vi "Agilent 34970 Set Switch.vi"(7 "Open/Close (F:Close)":bool, 8 "error in (no error)":errorcluster, 10 "Channel":string, 11 "VISA Refnum in":refnum<visa-resource-name>) -> (0 "error out":errorcluster, 1 "Success":bool, 2 "Channel State?":string, 3 "VISA Resource Name Out":refnum<visa-resource-name>)   [LabVIEW 2016]
uses:
  <vilib>/Utility/error.llb/whitespace.ctl
  Agilent 34970.lvlib
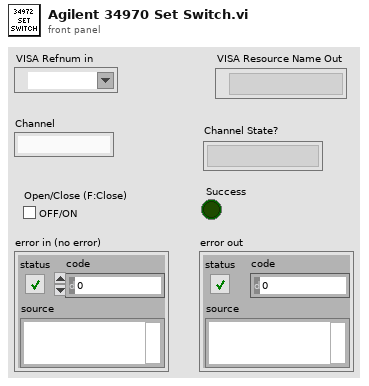
[diagram p1: front panel]
types:
  T1 = typedef "whitespace.ctl" = u16
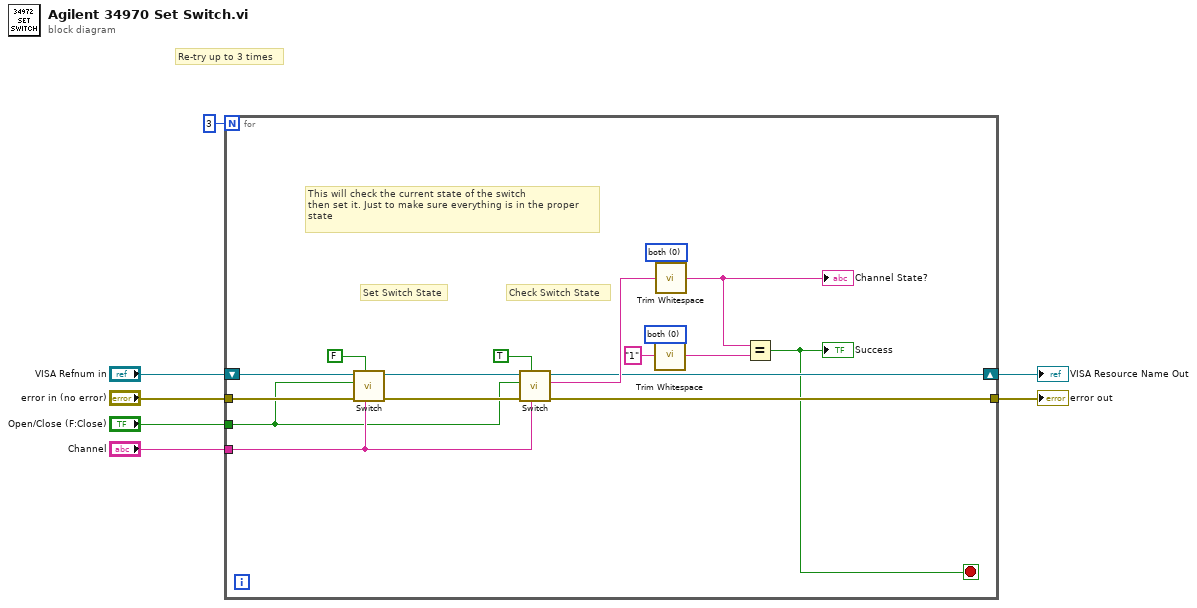
[diagram p0: block diagram]
diagram:
  # "Re-try up to 3 times"
  n1 = for {
    N: 3 -> [_]
    tunnel: "Channel" -> [w12]
    tunnel: "Open/Close (F:Close)" -> [w10]
    shift-right: [w9] -> w2
    shift-left: "VISA Refnum in" -> [w11]
    tunnel: "error in (no error)" -> [w15]
    tunnel: [w14] -> w6
    stop <- w8 stop-if-true
    w21 = T1 0 items=["both", "start of string", "end of string"] ("location (both)")
    w22 = T1 0 items=["both", "start of string", "end of string"] ("location (both)")
    # "This will check the current state of the switch\nthen set it. Just to make sure everything is in the proper\nstate"
    # "Set Switch State"
    # "Check Switch State"
    n2 = call "Switch.vi"("Channel List(empty)"=w12, "Set/Check (F:Set)"=FALSE, "error in (no error)"=w15, "Open/Close (F:Close)"=w10, "VISA Resource Name"=w11) -> ("error out"=w16:errorcluster, "VISA Resource Name Out"=w17:refnum<visa-resource-name>)  [unwired: 4 in, 1 out]
    n3 = call "Switch.vi"("Channel List(empty)"=w12, "Set/Check (F:Set)"=TRUE, "error in (no error)"=w16, "Open/Close (F:Close)"=w10, "VISA Resource Name"=w17) -> ("error out"=w14:errorcluster, "Channel State?"=w13:string, "VISA Resource Name Out"=w9:refnum<visa-resource-name>)  [unwired: 4 in]
    n4 = call <vilib>:"Trim Whitespace.vi"("string"="1", "location (both)"=w21) -> ("trimmed string"=w23:string)
    n5 = call <vilib>:"Trim Whitespace.vi"("string"=w13, "location (both)"=w22) -> ("trimmed string"=w20:string)
    "Channel State?" <- w20
    n6 = Equal?(x=w20, y=w23) -> (x = y?=w8:bool)
    "Success" <- w8
  }
  "error out" <- w6
  "VISA Resource Name Out" <- w2
